vi "Default Config--constant.vi"() -> (3 "Default Config":T1)   [LabVIEW 2020, in "VI Properties Editor.lvlib"]
doc: "Outputs the default config that will be used by the tool in the event that one or more config parameters are not found in the INI file."
uses:
  VI Properties Editor.lvlib
  CTLs/Config.ctl
  CTLs/Filter Info.ctl
  CTLs/Filter Column.ctl
  CTLs/Filter Type.ctl
  <vilib>/Utility/sysdir.llb/System Directory Type.ctl
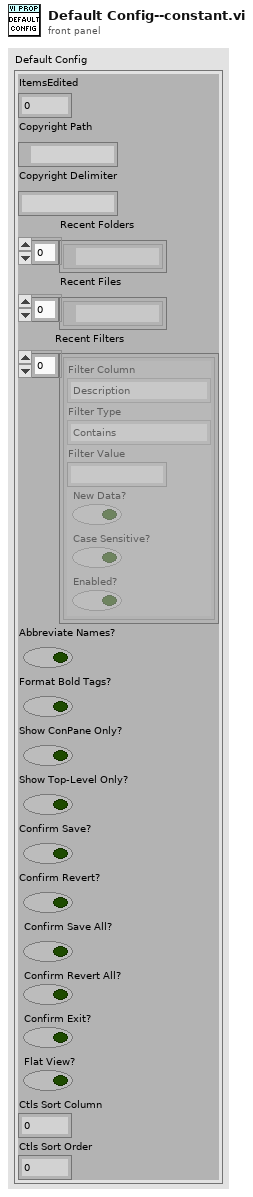
[diagram p1: front panel]
types:
  T1 = typedef "VI Properties Editor.lvlib/Config.ctl" = cluster{"ItemsEdited":u32, "Copyright Path":path, "Copyright Delimiter":string, "Recent Folders":path[], "Recent Files":path[], "Recent Filters":T2[], "Abbreviate Names?":bool, "Format Bold Tags?":bool, "Show ConPane Only?":bool, "Show Top-Level Only?":bool, "Confirm Save?":bool, "Confirm Revert?":bool, "Confirm Save All?":bool, "Confirm Revert All?":bool, "Confirm Exit?":bool, "Flat View?":bool, "Ctls Sort Column":i32, "Ctls Sort Order":i32}
  T2 = typedef "VI Properties Editor.lvlib/Filter Info.ctl" = cluster{"Filter Column":T3, "Filter Type":T4, "Filter Value":string, "New Data?":bool, "Case Sensitive?":bool, "Enabled?":bool}
  T3 = typedef "VI Properties Editor.lvlib/Filter Column.ctl" = enum16{"Name", "Path", "Type", "Window Title", "Description", "Help Path", "Help Tag", "Custom Title?", "Reentrancy", "Inlined?", "Help URL", "Help Type", "Allow Debugging?", "Auto Error Handling?", "Run When Opened?", "Suspend When Called?", "Priority", "Preferred Exec Sytem", "Control Label", "Control Caption", "Control Description", "Control Tip Strip"}
  T4 = typedef "VI Properties Editor.lvlib/Filter Type.ctl" = enum16{"Contains", "Equals", "Starts with", "Ends with", "Is empty", "Does not contain", "Does not equal", "Is not empty"}
  T5 = typedef "System Directory Type.ctl" = i32
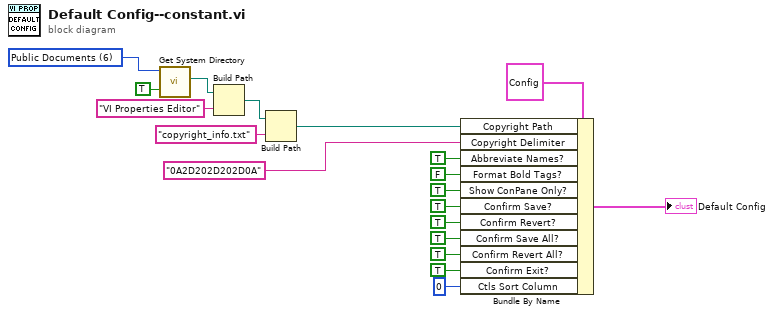
[diagram p0: block diagram]
diagram:
  w14 = T5 6 items=["User Home"=0, "User Desktop"=1, "User Documents"=2, "User Application Data"=3, "User Preferences"=4, "User Temporary"=5, "Public Documents"=6, "Public Application Data"=7, "Public Preferences"=8, "Public Cache"=13, "System Core Libraries"=9, "System Installed Libraries"=10, "Application Files"=11, "Boot Volume Root"=12] ("system directory type")
  n1 = call <vilib>:"Get System Directory.vi"("create directory if not found? (F)"=TRUE, "system directory type"=w14) -> ("system directory"=w16:path)  [unwired: 9 in]
  n2 = Build Path(base path=w16, name or relative path="VI Properties Editor") -> (appended path=w10:path)
  n3 = Build Path(base path=w10, name or relative path="copyright_info.txt") -> (appended path=w2:path)
  n4 = Bundle By Name(cluster=T1 {"ItemsEdited"=0, "Copyright Path"=path "", "Copyright Delimiter"="", "Recent Folders"=[], "Recent Files"=[], "Recent Filters"=[], "Abbreviate Names?"=FALSE, "Format Bold Tags?"=FALSE, "Show ConPane Only?"=FALSE, "Show Top-Level Only?"=FALSE, "Confirm Save?"=FALSE, "Confirm Revert?"=FALSE, "Confirm Save All?"=FALSE, "Confirm Revert All?"=FALSE, "Confirm Exit?"=FALSE, "Flat View?"=FALSE, "Ctls Sort Column"=0, "Ctls Sort Order"=0} ("Config"), "Copyright Path"=w2, "Copyright Delimiter"="0A2D202D202D0A" ("Hex String"), "Abbreviate Names?"=TRUE, "Format Bold Tags?"=FALSE ("View Formatted Bold"), "Show ConPane Only?"=TRUE, "Confirm Save?"=TRUE ("Show Save Dialog?"), "Confirm Revert?"=TRUE ("Show Revert Dialog?"), "Confirm Save All?"=TRUE ("Show Save All Dialog?"), "Confirm Revert All?"=TRUE ("Show Revert All Dialog?"), "Confirm Exit?"=TRUE, "Ctls Sort Column"=0) -> (→"Default Config":T1)
